vi "Connect.vi"(8 "error in (no error)":errorcluster, 11 "TCP_Client in":refnum<class "TCP_Client.lvclass">) -> (0 "error out":errorcluster, 3 "TCP_Client out":refnum<class "TCP_Client.lvclass">)   [LabVIEW 2023, in "TCP_Client.lvlib" / "TCP_Client.lvclass"]
uses:
  TCP_Client.lvclass
  <vilib>/ActorFramework/Actor/Actor.lvclass/Actor.ctl
  <vilib>/ActorFramework/Message Enqueuer/Message Enqueuer.lvclass/Message Enqueuer.ctl
  TCP_Client.lvclass/TCP_Client.ctl
  TCP_Client Messages/DisabelConnectButton Msg/DisabelConnectButton Msg.lvclass/DisabelConnectButton Msg.ctl
  <vilib>/ActorFramework/Message Enqueuer/Init from Existing Queue.vi
  <vilib>/ActorFramework/Message Enqueuer/Enqueue.vi
  TCP_Client Messages/LookForStartOfMessage Msg/LookForStartOfMessage Msg.lvclass
  TCP_Client Messages/DisabelConnectButton Msg/DisabelConnectButton Msg.lvclass
  TCP_Client Messages/Connect Msg/Connect Msg.lvclass
  <vilib>/ActorFramework/Stop Msg/Stop Msg.lvclass
  <vilib>/ActorFramework/Message Priority Queue/Priority Enqueue.vi
  <vilib>/ActorFramework/Message Enqueuer/Message Enqueuer.lvclass
  <vilib>/ActorFramework/Actor/Actor.lvclass
  C:/Program Files (x86)/National Instruments/LabVIEW 2023/vi.lib/ActorFramework/Actor/Actor.lvclass
  C:/Source/LabVIEW/TCP_server/TCP_Client/TCP_Client/TCP_Client.lvclass
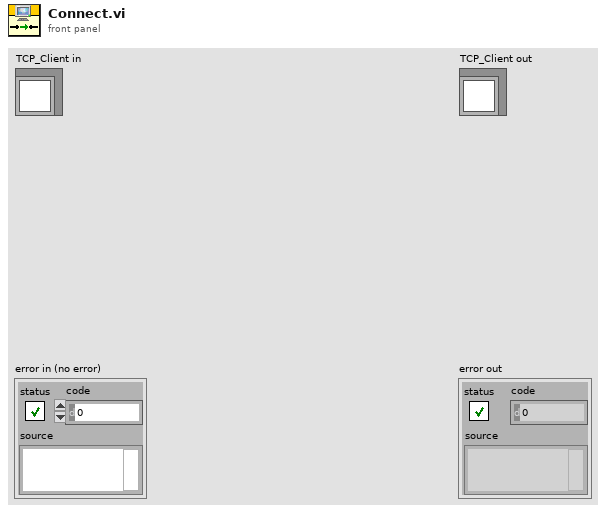
[diagram p1: front panel]
types:
  T1 = enum8{"Enabled", "Disabled", "Disabled and Grayed Out"}
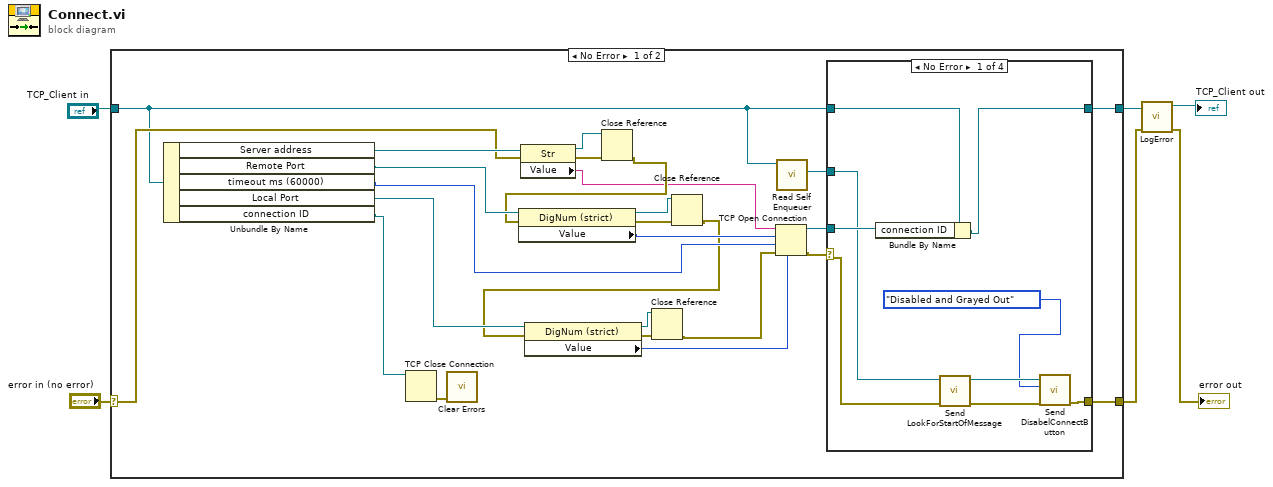
[diagram p0: block diagram]
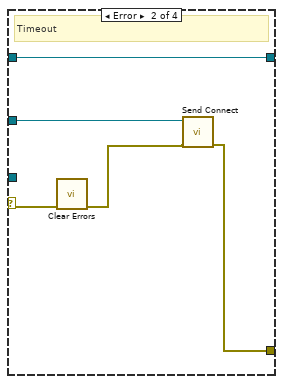
[diagram p2: hidden frame]
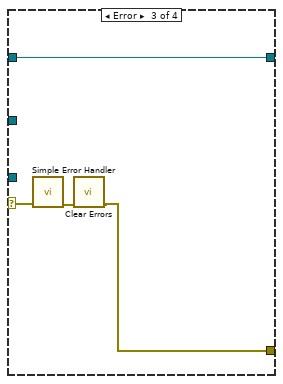
[diagram p3: hidden frame]
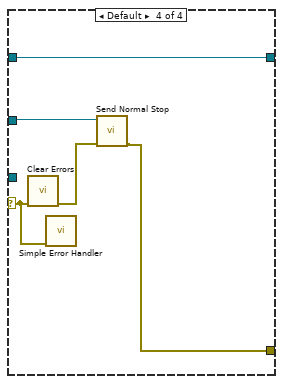
[diagram p4: hidden frame]
diagram:
  n1 = case shown="No Error" "error in (no error)" {
    selector: "error in (no error)" -> [w25 w56]
    tunnel: [w15 w56] -> w2
    tunnel: [w16 w55] -> w4
    tunnel: "TCP_Client in" -> [w17 w55]
    frame No Error {
      n2 = Unbundle By Name(w17) -> ("Server address"=w31:refnum<vi>, "Remote Port"=w30:refnum<vi>, "timeout ms (60000)"=w18:i32, "Local Port"=w14:refnum<vi>, "connection ID"=w8:refnum<k5>)
      n3 = TCP Close Connection(connection ID=w8) -> (error out=w7:errorcluster)  [unwired: 2 in, 1 out]
      n4 = call <vilib>:"Clear Errors.vi"("error in (no error)"=w7) -> ()  [unwired: 5 in, 2 out]
      n5 = property class="Str"(reference=w31, error in=w25) -> (reference out=w28:refnum<vi>, error out=w29:errorcluster, "Value"=w23:string)
      n6 = Close Reference(reference=w28, error in (no error)=w29) -> (error out=w24:errorcluster)
      n7 = property class="DigNum (strict)"(reference=w30, error in=w24) -> (reference out=w26:refnum<vi>, error out=w27:errorcluster, "Value"=w22:u16)
      n8 = Close Reference(reference=w26, error in (no error)=w27) -> (error out=w10:errorcluster)
      n9 = property class="DigNum (strict)"(reference=w14, error in=w10) -> (reference out=w11:refnum<vi>, error out=w12:errorcluster, "Value"=w13:u16)
      n10 = Close Reference(reference=w11, error in (no error)=w12) -> (error out=w9:errorcluster)
      n11 = TCP Open Connection(address=w23, remote port or service name=w22, timeout ms (60000)=w18, local port=w13, error in (no error)=w9) -> (connection ID=w20:refnum<k5>, error out=w21:errorcluster)
      n12 = call <vilib>:"Read Self Enqueuer.vi"("Actor"=w17) -> ("Self Enqueuer"=w19:refnum<class "Message Enqueuer.lvclass">)  [unwired: 10 in]
      n13 = case shown="No Error" w21 {
        selector: w21 -> [w36 w44 w48 w50]
        tunnel: w20 -> [w39 _ _ _]
        tunnel: w19 -> [w37 w43 _ w54]
        tunnel: w17 -> [w40 w45 w49 w51]
        tunnel: [w38 w45 w49 w51] -> w16
        tunnel: [w34 w41 w46 w53] -> w15
        frame No Error {
          n14 = Bundle By Name(cluster=w40, "connection ID"=w39) -> (w38:refnum<class "TCP_Client.lvclass">)
          n15 = call "Send LookForStartOfMessage.vi"("error in (no error)"=w36, "Message Enqueuer"=w37) -> ("error out"=w35:errorcluster, "Message Enqueuer out"=w33:refnum<class "Message Enqueuer.lvclass">)  [unwired: 8 in]
          n16 = call "Send DisabelConnectButton.vi"("error in (no error)"=w35, "Connect button Disabled"=T1."Disabled and Grayed Out", "Message Enqueuer"=w33) -> ("error out"=w34:errorcluster)  [unwired: 7 in, 1 out]
        }
        frame Error {
          # "Timeout"
          n17 = call <vilib>:"Clear Errors.vi"("error in (no error)"=w44) -> ("error out"=w42:errorcluster)  [unwired: 5 in, 1 out]
          n18 = call "Send Connect.vi"("error in (no error)"=w42, "Message Enqueuer"=w43) -> ("error out"=w41:errorcluster)  [unwired: 8 in, 1 out]
        }
        frame Error {
          n19 = call <vilib>:"Simple Error Handler.vi"("error in (no error)"=w48) -> ("error out"=w47:errorcluster)  [unwired: 4 in, 4 out]
          n20 = call <vilib>:"Clear Errors.vi"("error in (no error)"=w47) -> ("error out"=w46:errorcluster)  [unwired: 5 in, 1 out]
        }
        frame Default {
          n21 = call <vilib>:"Clear Errors.vi"("error in (no error)"=w50) -> ("error out"=w52:errorcluster)  [unwired: 5 in, 1 out]
          n22 = call <vilib>:"Simple Error Handler.vi"("error in (no error)"=w50) -> ()  [unwired: 4 in, 5 out]
          n23 = call <vilib>:"Send Normal Stop.vi"("error in (no error)"=w52, "Message Enqueuer"=w54) -> ("error out"=w53:errorcluster)  [unwired: 9 in]
        }
      }
    }
    frame Error {
    }
  }
  n24 = call "LogError.vi"("error in (no error)"=w2, "TCP_Client in"=w4) -> ("error out"=→"error out":errorcluster, "TCP_Client out"=→"TCP_Client out":refnum<class "TCP_Client.lvclass">)  [unwired: 8 in]
